vi "Геометр прогр.vi"() -> ()   [LabVIEW 2021]
panel:
  out "Сумма":dbl
  out "Array":dbl[](array[numeric])
  in  "Множитель":dbl
  in  "Первый\nчлен":dbl
  in  "Количество \nЭлеметнов":dbl
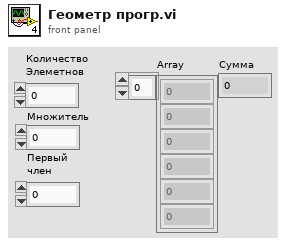
[diagram p1: front panel]
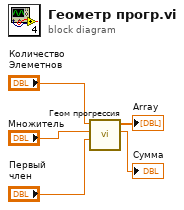
[diagram p0: block diagram]
diagram:
  n1 = call "Геом прогрессия.vi"("Первый\nчлен"="Первый\nчлен", "Множитель"="Множитель", "Количество \nЭлеметнов"="Количество \nЭлеметнов") -> ("Сумма"=→"Сумма":dbl, "Array"=→"Array":dbl[])  [unwired: 7 in]
